vi "Get Active ProjectPath.vi"(11 "error in (no error)":errorcluster) -> (4 "Project Path":path, 15 "error out":errorcluster)   [LabVIEW 2021, in "Packager Helpers.lvlib"]
uses:
  Packager Helpers.lvlib
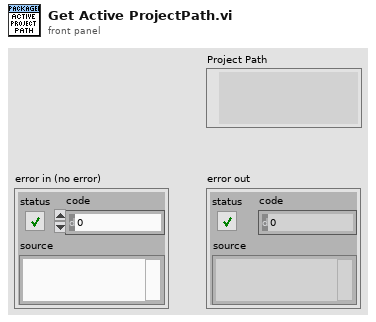
[diagram p1: front panel]
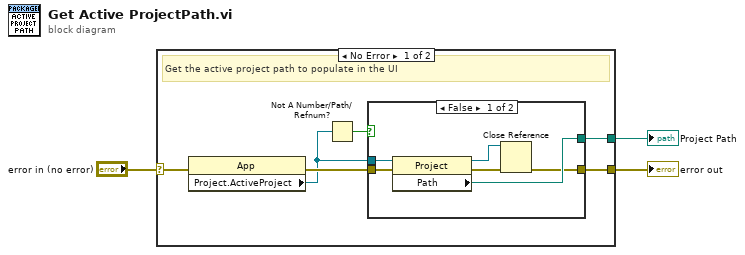
[diagram p0: block diagram]
diagram:
  n1 = case shown="No Error" "error in (no error)" {
    selector: "error in (no error)" -> [w9 w17]
    tunnel: [w7 _] -> w3
    tunnel: [w4 w17] -> w1
    frame No Error {
      # "Get the active project path to populate in the UI"
      n2 = property class="App"(error in=w9) -> (error out=w8:errorcluster, "Project.ActiveProject"=w6:refnum<vi>)  [unwired: 1 in, 1 out]
      n3 = Not A Number/Path/Refnum?(number/path/refnum=w6) -> (NaN/Path/Refnum?=w5:bool)
      n4 = case shown="False" w5 {
        tunnel: w8 -> [w15 w16]
        tunnel: [w12 _] -> w7
        tunnel: w6 -> [w13 _]
        tunnel: [w10 w16] -> w4
        frame False {
          n5 = property class="Project"(reference=w13, error in=w15) -> (reference out=w14:refnum<vi>, error out=w11:errorcluster, "Path"=w12:path)
          n6 = Close Reference(reference=w14, error in (no error)=w11) -> (error out=w10:errorcluster)
        }
        frame True {
        }
      }
    }
    frame Error {
    }
  }
  "error out" <- w1
  "Project Path" <- w3
